vi "Get Record Info.vi"(8 "error in":errorcluster, 11 "FPGA VI Reference In":refnum<k20>) -> (0 "error out":errorcluster, 1 "Record Length":u32, 2 "Records to Acquire":u32, 3 "FPGA VI Reference Out":refnum<k20>, 4 "Num of Channels":u32)   [LabVIEW 2011]
uses:
  <vilib>/Utility/error.llb/Error Cluster From Error Code.vi
  <vilib>/rvi/errors/niLvFpgaAdjustHostInterfaceError.vi
  <vilib>/rvi/interface/nirviReadWriteControl/nirviReadWriteControl.xnode
  NiFpgaLv.dll
  <vilib>/rvi/interface/Simulation/niFpgaSimulationCallBeginRW.vi
panel:
  out "Post Trigger Samples":u32
  out "Pre Trigger Samples":u32
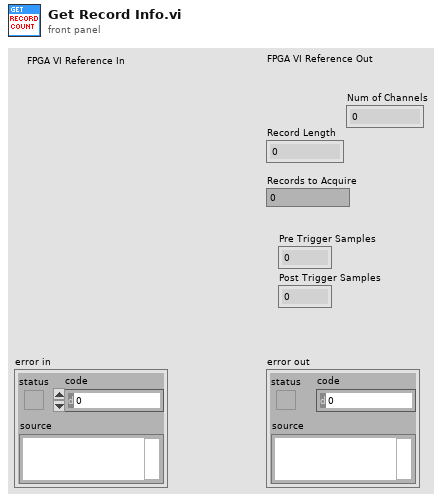
[diagram p1: front panel]
types:
  T1 = cluster{"Load Record Parameters?":bool, "Pre Trigger Samples":u32, "Post Trigger Samples":u32, "Trigger Hold Off":u32, "Record Count":u32}
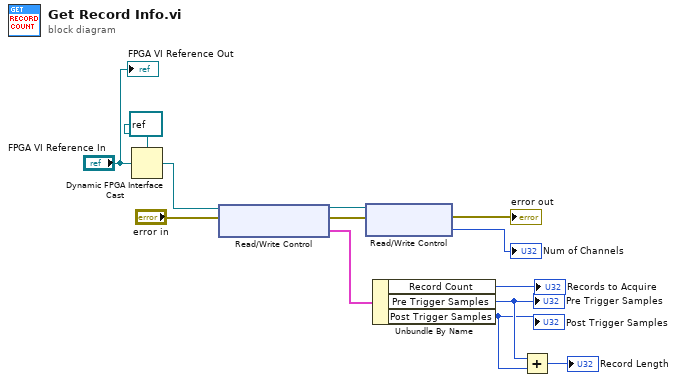
[diagram p0: block diagram]
diagram:
  n1 = Dynamic FPGA Interface Cast(Session In=refnum<k20> refnum ("Type"), Type="FPGA VI Reference In") -> (Session Out=w11:refnum<k20>)
  n2 = xnode "Read/Write Control"("FPGA VI Reference In"=w11, "error in"="error in") -> ("FPGA VI Reference Out"=w4:refnum<k20>, "error out"=w3:errorcluster, "Record Parameters"=w9:T1)
  n3 = xnode "Read/Write Control"("FPGA VI Reference In"=w4, "error in"=w3) -> ("error out"=→"error out":errorcluster, "Num Channels"=→"Num of Channels":u32)  [unwired: 1 out]
  n4 = Unbundle By Name(w9) -> ("Record Count"=→"Records to Acquire":u32, "Pre Trigger Samples"=w7:u32, "Post Trigger Samples"=w6:u32)
  "Pre Trigger Samples" <- w7
  "Post Trigger Samples" <- w6
  n5 = Add(x=w7, y=w6) -> (x+y=→"Record Length":u32)
  "FPGA VI Reference Out" <- "FPGA VI Reference In"
